vi "Set_Parameter_Instrument (Json).vi"(8 "error in (no error)":errorcluster caption="entrée d'erreur (pas d'erreur)", 10 "Parameter (Json)":string, 11 "Delay en entrée":refnum<class "Delay.lvclass">) -> (0 "error out":errorcluster caption="sortie d'erreur", 3 "Delay en sortie":refnum<class "Delay.lvclass">)   [LabVIEW 2020, in "Library Test.lvlib" / "Delay.lvclass"]
uses:
  Delay.lvclass
  C:/Users/ngarcin/OneDrive - Altyor/Standard TB/Class/Test/Test (Default)/Test (Default).lvclass
  Delay.lvclass/Delay.ctl
  JSON API/JSON Value/Set from JSON string.vi
  Test_Without_Instr/Test_Without_Inst.lvclass
  JSON API/JSON Value/JSON Value.lvclass
  JSON API/Variant JSON/Variant JSON.lvlib
  JSON API/Get Polymorphic/JSON GetSet.lvlib
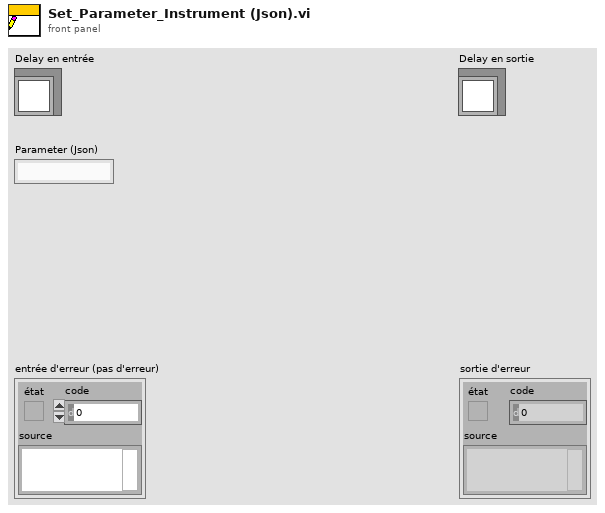
[diagram p1: front panel]
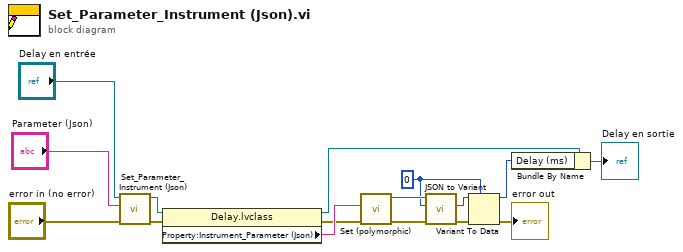
[diagram p0: block diagram]
diagram:
  w9 = u32 0 ("Channel")
  n1 = call-parent "Set_Parameter_Instrument (Json).vi"("error in (no error)"="error in (no error)", "Parameter (Json)"="Parameter (Json)", "Test (Default) en entrée"="Delay en entrée") -> ("error out"=w4:errorcluster, "Test (Default) en sortie"=w6:refnum<class "Delay.lvclass">)  [unwired: 7 in]
  n2 = property class="Delay.lvclass"(reference=w6, error in=w4) -> (reference out=w2:refnum<class "Delay.lvclass">, error out=w7:errorcluster, "Property:Instrument_Parameter (Json)"=w8:string)
  n3 = call-poly "Set (polymorphic).vi"("error in (no error)"=w7, "JSON stream"=w8) -> ("error out"=w11:errorcluster, "JSON Value out"=w13:refnum<class "JSON Value.lvclass">)  [unwired: 7 in, 1 out]
  n4 = call "JSON to Variant.vi"("error in (no error)"=w11, "Variant (Data Type)"=w9, "JSON Value"=w13) -> ("error out"=w12:errorcluster, "Variant out"=w10:variant)  [unwired: 7 in]
  n5 = Variant To Data(error in=w12, type=w9, Variant=w10) -> (data=w1:u32, error out=→"error out":errorcluster)
  n6 = Bundle By Name(cluster=w2, "Delay (ms)"=w1) -> (→"Delay en sortie":refnum<class "Delay.lvclass">)
